vi "Handle Anomaly Log.vi"(0 "Data":dbl[][](array[numeric]), 1 "FPGAnomalies":i32[](array[numeric]), 3 "Init Anomalies":i32[](array[numeric]), 5 "Enable":bool, 7 "RowCount In":i32, 9 "Anomaly Log Path":path, 11 "Current Data Path":path) -> ()   [LabVIEW 2018]
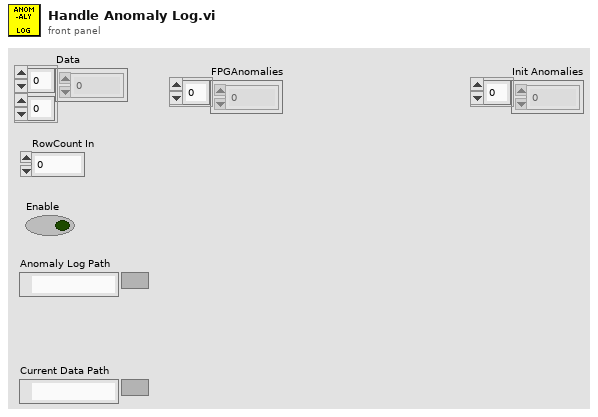
[diagram p1: front panel]
types:
  T1 = enum16{"open", "replace", "create", "open or create", "replace or create", "replace or create with confirmation"}
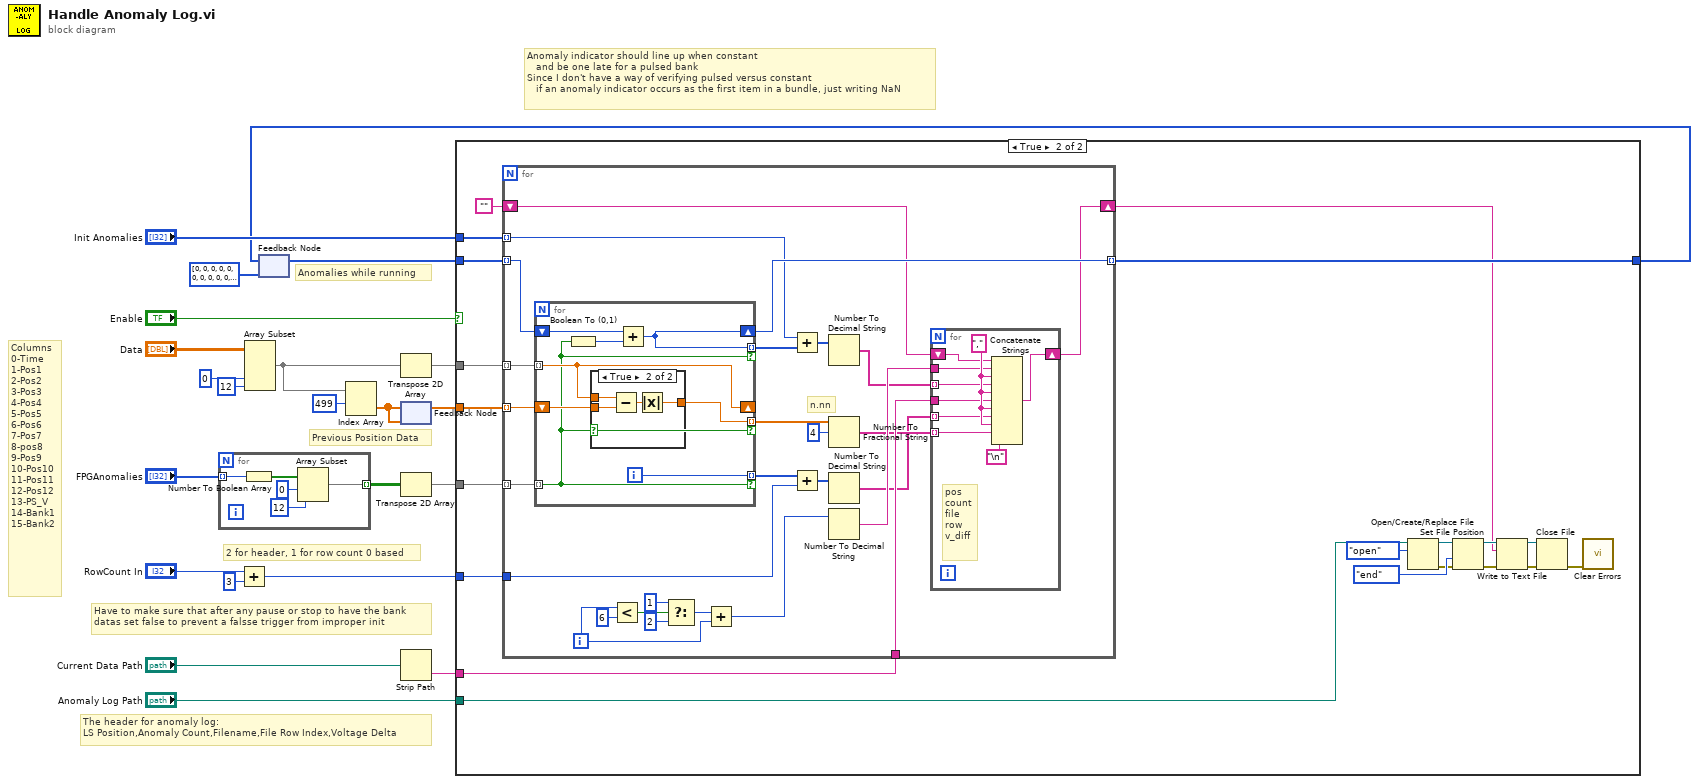
[diagram p0: block diagram]
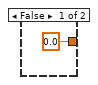
[diagram p3: hidden frame]
diagram:
  # "Anomaly indicator should line up when constant\n   and be one late for a pulsed bank\nSince I don't have a way of verifying pulsed versus constant\n   if an anomaly indicator occurs as the first item in a bundle, just writing NaN"
  # "Anomalies while running"
  # "Have to make sure that after any pause or stop to have the bank\ndatas set false to prevent a falsse trigger from improper init"
  # "Previous Position Data"
  # "2 for header, 1 for row count 0 based"
  # "The header for anomaly log:\nLS Position,Anomaly Count,Filename,File Row Index,Voltage Delta"
  # "Columns\n0-Time\n1-Pos1\n2-Pos2\n3-Pos3\n4-Pos4\n5-Pos5\n6-Pos6\n7-Pos7\n8-pos8\n9-Pos9\n10-Pos10\n11-Pos11\n12-Pos12\n13-PS_V\n14-Bank1\n15-Bank2"
  n1 = for {
    tunnel: "FPGAnomalies" -> [w27] mode=indexing
    tunnel: [w23] -> w6 mode=indexing
    n2 = Number To Boolean Array(number=w27) -> (Boolean array=w26:bool[])
    n3 = Array Subset(array=w26, index=0, length=12) -> (w23:bool[])
  }
  n4 = Add(x="RowCount In", y=3 ("x")) -> (x+y=w18:i32)
  n5 = Array Subset(array="Data", index (col)=0 ("index"), length (col)=12 ("length")) -> (w13:dbl[][])  [unwired: 2 in]
  n6 = feedback #1(i32[] [0, 0, 0, 0, 0, 0, 0, 0, 0, 0, 0, 0]) -> (w2:i32[])
  n7 = Index Array(array=w13, index (row)=499) -> (element=w15:dbl[])  [unwired: 1 in]
  n8 = Transpose 2D Array(2D array=w13) -> (transposed array=w19:dbl[][])
  n9 = feedback #2(w15) -> (w12:dbl[])
  n10 = feedback-in #2(w15) -> ()
  n11 = Transpose 2D Array(2D array=w6) -> (transposed array=w5:bool[][])
  n12 = Strip Path(path="Current Data Path") -> (name=w8:string)  [unwired: 1 out]
  n13 = case shown="True" "Enable" {
    tunnel: w19 -> [_ w48]
    tunnel: w18 -> [_ w47]
    tunnel: w8 -> [_ w46]
    tunnel: "Anomaly Log Path" -> [_ w34]
    tunnel: w12 -> [_ w36]
    tunnel: w5 -> [_ w35]
    tunnel: "Init Anomalies" -> [_ w33]
    tunnel: w2 -> [w28 w32]
    tunnel: [w28 w31] -> w1
    frame False {
    }
    frame True {
      n14 = for {
        tunnel: w48 -> [w70] mode=indexing
        tunnel: w36 -> [w71] mode=indexing
        tunnel: w47 -> [w63]
        tunnel: w46 -> [w52]
        tunnel: w35 -> [w68] mode=indexing
        tunnel: w33 -> [w58] mode=indexing
        tunnel: w32 -> [w62] mode=indexing
        tunnel: [w61] -> w31 mode=indexing
        shift-right: [w54] -> w29
        shift-left: "" -> [w55]
        i -> [w57]
        # "n.nn"
        n15 = for {
          tunnel: w70 -> [w92] mode=indexing
          shift-right: [w92] -> _
          shift-left: w71 -> [w91]
          tunnel: w68 -> [w85] mode=indexing
          tunnel: [w86] -> w66 mode=indexing if=w85
          tunnel: [w90] -> w56 mode=indexing if=w85
          shift-right: [w87] -> w61
          shift-left: w62 -> [w89]
          tunnel: [w87] -> w60 mode=indexing if=w85
          i -> [w90]
          n16 = Boolean To (0,1)(Boolean=w85) -> (0, 1=w88:i16)
          n17 = case shown="True" w85 {
            tunnel: w92 -> [_ w97]
            tunnel: w91 -> [_ w96]
            tunnel: [0.0 w94] -> w86
            frame False {
            }
            frame True {
              n18 = Subtract(x=w97, y=w96) -> (x-y=w95:dbl)
              n19 = Absolute Value(x=w95) -> (abs(x)=w94:dbl)
            }
          }
          n20 = Add(x=w89, y=w88) -> (x+y=w87:i32)
        }
        n21 = Less?(x=w57, y=6) -> (x < y?=w74:bool)
        n22 = Select(t=1 ("index"), s=w74, f=2 ("index")) -> (s? t:f=w69:i32)
        n23 = Add(x=w69, y=w57) -> (x+y=w64:i32)
        n24 = Add(x=w58, y=w60) -> (x+y=w59:i32[])
        n25 = Add(x=w56, y=w63) -> (x+y=w65:i32[])
        n26 = Number To Decimal String(number=w59) -> (decimal integer string=w51:string[])  [unwired: 1 in]
        n27 = Number To Fractional String(number=w66, width (-)=i16 4) -> (F-format string=w50:string[])  [unwired: 2 in]
        n28 = Number To Decimal String(number=w65) -> (decimal integer string=w49:string[])  [unwired: 1 in]
        n29 = Number To Decimal String(number=w64) -> (decimal integer string=w53:string)  [unwired: 1 in]
        n30 = for {
          shift-right: [w81] -> w54
          shift-left: w55 -> [w82]
          tunnel: w53 -> [w80]
          tunnel: w52 -> [w79]
          tunnel: w51 -> [w78] mode=indexing
          tunnel: w50 -> [w77] mode=indexing
          tunnel: w49 -> [w76] mode=indexing
          w83 = ","
          # "pos\ncount\nfile\nrow\nv_diff"
          n31 = Concatenate Strings(w82, w80, w83, w78, w83, w79, w83, w76, w83, w77, "\n") -> (w81:string)
        }
      }
      n32 = Open/Create/Replace File(file path (use dialog)=w34, operation (0:open)=T1."open") -> (refnum out=w41:refnum<file>, error out=w42:errorcluster)  [unwired: 4 in, 1 out]
      n33 = Set File Position(refnum=w41, from (0:start)=enum16{"start", "end", "current"}."end", error in=w42) -> (refnum out=w44:refnum<file>, error out=w45:errorcluster)  [unwired: 1 in]
      n34 = Write to Text File(file (use dialog)=w44, text=w29, error in=w45) -> (refnum out=w38:refnum<file>, error out=w37:errorcluster)  [unwired: 1 in, 1 out]
      n35 = Close File(refnum=w38, error in=w37) -> (error out=w39:errorcluster)  [unwired: 1 out]
      n36 = call <vilib>:"Clear Errors.vi"("error in (no error)"=w39) -> ()  [unwired: 5 in, 2 out]
    }
  }
  n37 = feedback-in #1(w1) -> ()
